vi "sortInternalEvents.vi"(8 "error in (no error)":errorcluster, 11 "ScriptEventList in":refnum<class "ScriptEventList.lvclass">) -> (0 "error out":errorcluster, 3 "ScriptEventList out":refnum<class "ScriptEventList.lvclass">)   [LabVIEW 2011, in "Tools.lvlib" / "Scripting.lvlib" / "ScriptEventList.lvclass"]
uses:
  ScriptEventList.lvclass
  ScriptEventList.lvclass/ScriptEventList.ctl
  ScriptEvent.lvclass
  DatabaseHelpers/Database Objects/Channel/Channel.lvclass
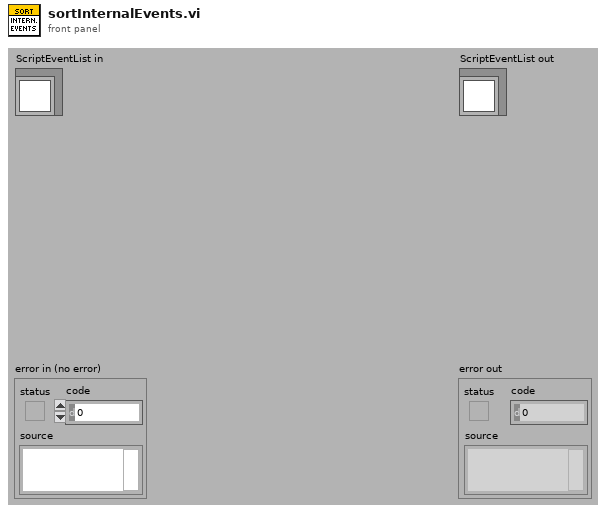
[diagram p1: front panel]
types:
  T1 = cluster{"time":dbl, dbl, "channel_name":string, i32}
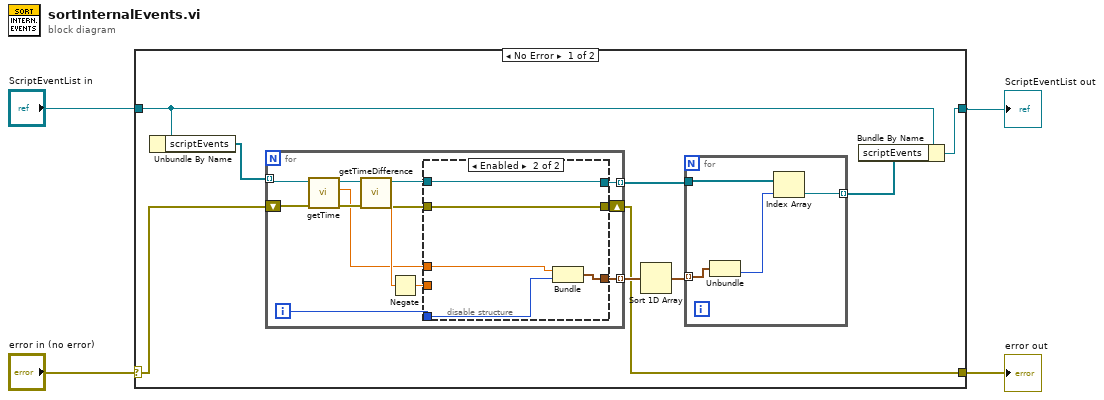
[diagram p0: block diagram]
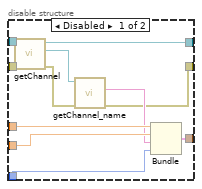
[diagram p2: hidden frame]
diagram:
  n1 = case shown="No Error" "error in (no error)" {
    selector: "error in (no error)" -> [w7 w48]
    tunnel: [w10 w48] -> w1
    tunnel: [w8 w47] -> w2
    tunnel: "ScriptEventList in" -> [w5 w47]
    frame No Error {
      n2 = Unbundle By Name(w5) -> ("scriptEvents"=w6:refnum<class "ScriptEvent.lvclass">[])
      n3 = for {
        tunnel: w6 -> [w30] mode=indexing
        shift-right: [w19] -> w10
        shift-left: w7 -> [w29]
        tunnel: [w20] -> w13 mode=indexing
        tunnel: [w18] -> w11 mode=indexing
        i -> [w21]
        n4 = call "getTime.vi"("error in (no error)"=w29, "ScriptEvent.lvclass in"=w30) -> ("error out"=w27:errorcluster, "time"=w23:dbl, "ScriptEvent.lvclass out"=w28:refnum<class "ScriptEvent.lvclass">)  [unwired: 7 in]
        n5 = call "getTimeDifference.vi"("error in (no error)"=w27, "ScriptEvent.lvclass in"=w28) -> ("error out"=w25:errorcluster, "time difference"=w26:dbl, "ScriptEvent.lvclass out"=w24:refnum<class "ScriptEvent.lvclass">)  [unwired: 7 in]
        n6 = Negate(x=w26) -> (-x=w22:dbl)
        n7 = disable-structure shown="Enabled" {
          disable-tunnel: w25 -> [w41 w45]
          disable-tunnel: w24 -> [w40 w46]
          disable-tunnel: w23 -> [w37 w44]
          disable-tunnel: w22 -> [w36 _]
          disable-tunnel: w21 -> [w34 w43]
          disable-tunnel: [w33 w42] -> w20
          disable-tunnel: [w32 w45] -> w19
          disable-tunnel: [w31 w46] -> w18
          frame Disabled {
            n8 = call-dynamic "getChannel.vi"("error in (no error)"=w41, "ScriptEvent.lvclass in"=w40) -> ("error out"=w38:errorcluster, "Channel.lvclass"=w39:refnum<class "Channel.lvclass">, "ScriptEvent.lvclass out"=w31:refnum<class "ScriptEvent.lvclass">)  [unwired: 7 in]
            n9 = call "getChannel_name.vi"("error in (no error)"=w38, "Channel.lvclass in"=w39) -> ("error out"=w32:errorcluster, "channel_name"=w35:string)  [unwired: 7 in, 1 out]
            n10 = Bundle("time"=w37, w36, "channel_name"=w35, w34) -> (w33:T1)  [unwired: 1 in]
          }
          frame Enabled {
            n11 = Bundle("time"=w44, w43) -> (w42:cluster{"time":dbl, i32})  [unwired: 1 in]
          }
        }
      }
      n12 = Sort 1D Array(array=w13) -> (sorted array=w12:cluster{"time":dbl, i32}[])
      n13 = for {
        tunnel: w12 -> [w16] mode=indexing
        tunnel: w11 -> [w17]
        tunnel: [w15] -> w9 mode=indexing
        n14 = Unbundle(w16) -> (w14:i32)  [unwired: 1 out]
        n15 = Index Array(array=w17, index=w14) -> (element=w15:refnum<class "ScriptEvent.lvclass">)
      }
      n16 = Bundle By Name(cluster=w5, "scriptEvents"=w9) -> (w8:refnum<class "ScriptEventList.lvclass">)
    }
    frame Error {
    }
  }
  "error out" <- w1
  "ScriptEventList out" <- w2
